vi "Init.vi"(8 "error in (no error)":errorcluster, 11 "reference in":refnum<class "Switch_MotorP5.lvclass">) -> (0 "error out":errorcluster, 3 "reference out":refnum<class "Switch_MotorP5.lvclass">)   [LabVIEW 2022 SP3, in "Switch_MotorP5.lvlib" / "Switch_MotorP5.lvclass"]
uses:
  Switch_MotorP5.lvclass
  <vilib>/Instr/_visa.llb/VISA Configure Serial Port (Instr).vi
  Components/SwitchBase.lvlibp/SwitchBase.lvclass
  Components/ViPER.lvlibp/ViPER.lvclass
  C:/Projects/Medulla/ViPER/Examples/Flux_Capacitor_Tester/Components/ViPER.lvlibp/ViPER.lvclass
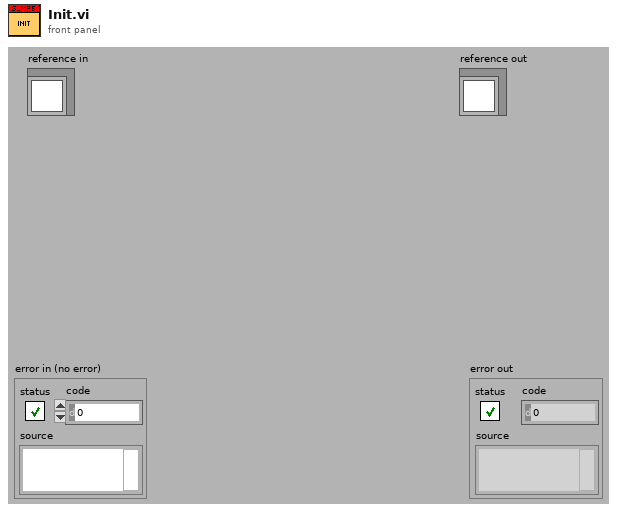
[diagram p1: front panel]
types:
  T1 = enum32{"M1", "M2", "M3", "M4", "M5", "M6", "M7", "M8"}
  T2 = typedef "Switch_MotorP5.lvlib/Switch_MotorP5.lvclass/ObjectAttributes.ctl" = cluster{"Config":T3, "VISA":refnum<visa-resource-name>, "RPM":i32, "States":bool[], "UpdateEvent":refnum<user-event>, "Motor":enum32{"M1", "M2", "M3", "M4", "M5", "M6", "M7", "M8"}}
  T3 = typedef "Switch_MotorP5.lvlib/Switch_MotorP5.lvclass/Config.ctl" = cluster{"COM":refnum<visa-resource-name>, "SwitchMap":cluster{"Name":string, "Description":string, "Group":string, "IsGroup":bool, "Motor":enum32{"M1", "M2", "M3", "M4", "M5", "M6", "M7", "M8", "NA"}}[], "Sim":bool}
  T4 = cluster{"Name":string, "Description":string, "Group":string, "IsGroup":bool, "Motor":enum32{"M1", "M2", "M3", "M4", "M5", "M6", "M7", "M8", "NA"}}[]
  T5 = enum32{"M1", "M2", "M3", "M4", "M5", "M6", "M7", "M8", "NA"}
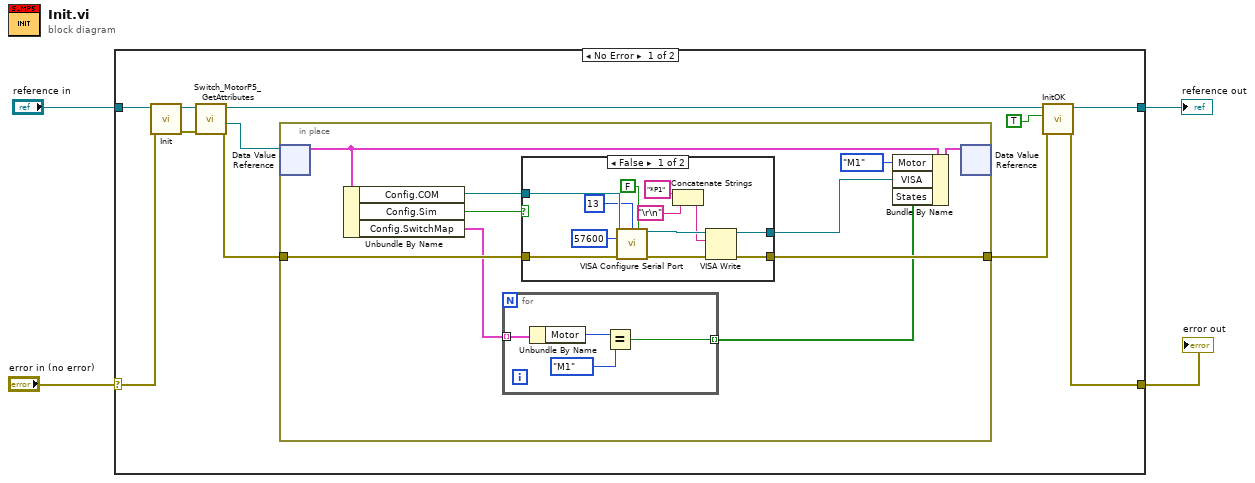
[diagram p0: block diagram]
diagram:
  n1 = case shown="No Error" "error in (no error)" {
    selector: "error in (no error)" -> [w14 w44]
    tunnel: [w5 w44] -> w3
    tunnel: [w8 w43] -> w1
    tunnel: "reference in" -> [w15 w43]
    frame No Error {
      n2 = call-parent "Init.vi"("error in (no error)"=w14, "reference in"=w15) -> ("error out"=w12:errorcluster, "reference out"=w13:refnum<class "Switch_MotorP5.lvclass">)  [unwired: 8 in]
      n3 = call "Switch_MotorP5_GetAttributes.vi"("error in (no error)"=w12, "reference in"=w13) -> ("error out"=w10:errorcluster, "DataRef"=w11:refnum<data-value>, "reference out"=w9:refnum<class "Switch_MotorP5.lvclass">)  [unwired: 6 in, 1 out]
      n4 = in-place {
        in-place-border: w10 -> [w25]
        in-place-border: [w21] -> w6
        n5 = in-place-dvr #1(w11) -> (w23:T2)  [unwired: 1 out]
        n6 = Unbundle By Name(w23) -> ("Config.COM"=w24:refnum<visa-resource-name>, "Config.Sim"=w19:bool, "Config.SwitchMap"=w18:T4)
        n7 = for {
          tunnel: w18 -> [w29] mode=indexing
          tunnel: [w27] -> w17 mode=indexing
          n8 = Unbundle By Name(w29) -> ("Motor"=w28:T5)
          n9 = Equal?(x=w28, y=T1."M1") -> (x = y?=w27:bool)
        }
        n10 = case shown="False" w19 {
          tunnel: w25 -> [w41 w42]
          tunnel: w24 -> [w40 _]
          tunnel: [w37 w42] -> w21
          tunnel: [w35 _] -> w20
          frame False {
            n11 = call-poly "VISA Configure Serial Port"("VISA resource name"=w40, "termination char\n(0xA = '\\n' = LF)"=u8 13 ("termination char\n(0xA = '\\n' = LF)"), "Enable Termination\nChar (T)"=FALSE ("Enable Termination\nChar (T)"), "baud rate (9600)"=u32 57600, "error in (no error)"=w41) -> ("VISA resource name out"=w36:refnum<visa-resource-name>, "error out"=w38:errorcluster)  [unwired: 9 in]
            n12 = Concatenate Strings("*P1", "\r\n") -> (w32:string)
            n13 = VISA Write(VISA resource name=w36, write buffer=w32, error in (no error)=w38) -> (VISA resource name out=w35:refnum<visa-resource-name>, error out=w37:errorcluster)  [unwired: 1 out]
          }
          frame True {
          }
        }
        n14 = Bundle By Name(cluster=w23, "Motor"=T1."M1", "VISA"=w20, "States"=w17) -> (w22:T2)
        n15 = in-place-dvr #1(w22) -> ()  [unwired: 2 out]
      }
      n16 = call "InitOK.vi"("error in (no error)"=w6, "Init OK?"=TRUE, "reference in"=w9) -> ("error out"=w5:errorcluster, "reference out"=w8:refnum<class "Switch_MotorP5.lvclass">)  [unwired: 7 in]
    }
    frame Error {
    }
  }
  "error out" <- w3
  "reference out" <- w1
